vi "LakeShore218_format_data.vi"(8 "name_array":string[](array[string]), 9 "value_array":dbl[](array[numeric]), 11 "time":timestamp) -> (1 "value_array_out":dbl[](array[numeric]), 3 "waveform_array":waveform(dbl)[](array[waveform])=[{"t0"=timestamp(0 s since 1904-01-01), "dt"=1.0, "Y"=[]}, {"t0"=timestamp(3732035173.078092 s since 1904-01-01), "dt"=1.0, "Y"=[302.8589782714844], "attributes"=variant("NI_ChannelName"=variant(string "T1"))}])   [LabVIEW 2019]
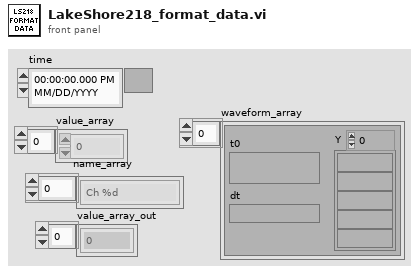
[diagram p1: front panel]
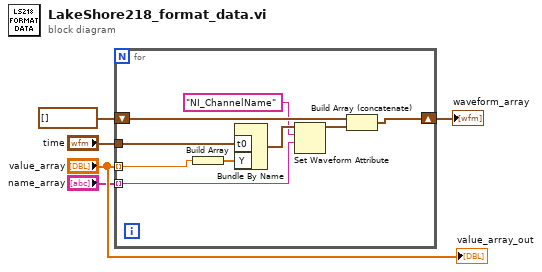
[diagram p0: block diagram]
diagram:
  n1 = for {
    tunnel: "time" -> [w12]
    tunnel: "value_array" -> [w10] mode=indexing
    shift-right: [w11] -> w3
    shift-left: waveform(dbl)[] [] -> [w14]
    tunnel: "name_array" -> [w6] mode=indexing
    n2 = Build Array(w10) -> (w13:dbl[])
    n3 = Bundle By Name("t0"=w12, "Y"=w13) -> (w8:waveform(dbl))  [unwired: 1 in]
    n4 = Set Waveform Attribute(5:w6, 6:"NI_ChannelName" ("name"), 7:w8) -> (3:w9:waveform(dbl))  [unwired: 1 in, 2 out]
    n5 = Build Array (concatenate)(w14, w9) -> (w11:waveform(dbl)[])
  }
  "waveform_array" <- w3
  "value_array_out" <- "value_array"
